vi "Apply special move.vi"(8 "error in (no error)":errorcluster, 10 "Position in":refnum<class "Position.lvclass">, 11 "enPassant in":refnum<class "enPassant.lvclass">) -> (0 "error out":errorcluster, 2 "Position out":refnum<class "Position.lvclass">, 3 "enPassant out":refnum<class "enPassant.lvclass">)   [LabVIEW 2015, in "Chesslib.lvlib" / "enPassant.lvclass"]
uses:
  enPassant.lvclass
  Move/Move.lvclass
  Position/Position.lvclass
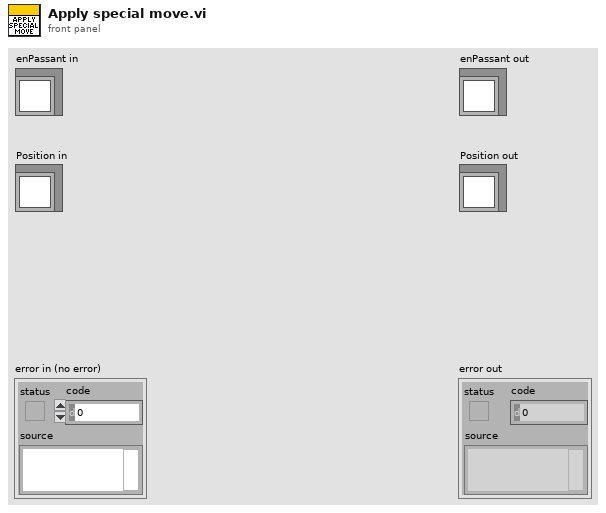
[diagram p1: front panel]
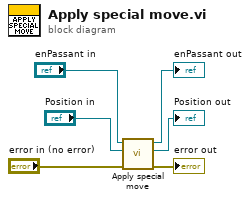
[diagram p0: block diagram]
diagram:
  n1 = call-parent "Apply special move.vi"("error in (no error)"="error in (no error)", "Position in"="Position in", "Move in"="enPassant in") -> ("error out"=→"error out":errorcluster, "Position out"=→"Position out":refnum<class "Position.lvclass">, "Move out"=→"enPassant out":refnum<class "enPassant.lvclass">)  [unwired: 6 in]
